vi "ConfigFile_ErrorHandler.vi"(8 "errorArray":errorcluster[](array[cluster]), 9 "foundArray":bool[](array[boolean]), 10 "configItemNameArray":string[](array[string]), 11 "configFilePath (No Path)":path=path "No Path") -> (0 "error out":errorcluster)   [LabVIEW 2024]
doc: "This VI handles errors from reading or writing a configuration file. <B>configFilePath</B> is the path to the configuration file. For the input arrays, all elements must correspond with each other. For example, <B>configItemNameArray[0]</B> is the name of the first configuration item. <B>foundArray[0]</B> is TRUE if the first configuration item was found. <B>errorArray[0]</B> has an error if the read operation for the first configuration item raised an error. <B>error out</B> concatenates all the errors for the configuration arrays into a single error structure."
panel:
  in  "errorCode (9999)":i32=9999
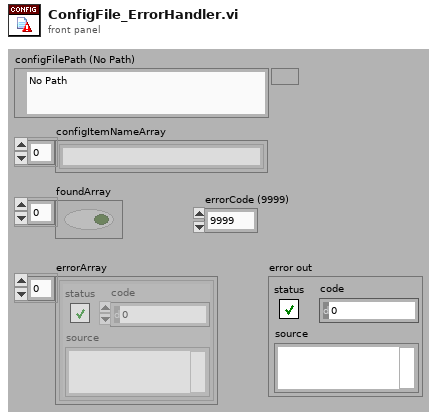
[diagram p1: front panel]
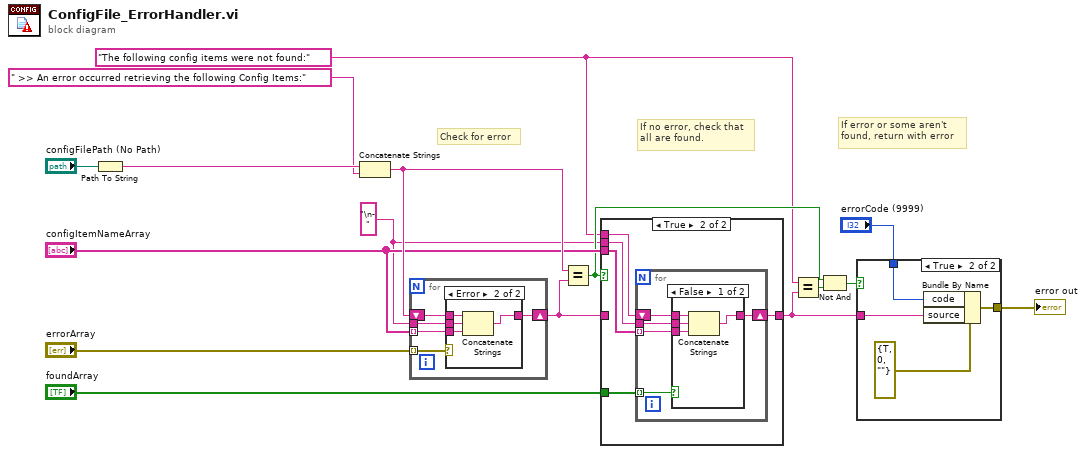
[diagram p0: block diagram]
diagram:
  w6 = "The following config items were not found:"
  w2 = "\n- "
  # "If no error, check that\nall are found."
  # "If error or some aren't\nfound, return with error"
  # "Check for error"
  n1 = Path To String(path="configFilePath (No Path)") -> (string=w15:string)
  n2 = Concatenate Strings(w15, " >> An error occurred retrieving the following Config Items:") -> (w13:string)
  n3 = for {
    tunnel: "errorArray" -> [w21] mode=indexing
    tunnel: "configItemNameArray" -> [w17] mode=indexing
    shift-right: [w20] -> w4
    shift-left: w13 -> [w19]
    tunnel: w2 -> [w18]
    n4 = case shown="Error" w21 {
      tunnel: [w22 w23] -> w20
      tunnel: w19 -> [w22 w26]
      tunnel: w18 -> [_ w25]
      tunnel: w17 -> [_ w24]
      frame No Error {
      }
      frame Error {
        n5 = Concatenate Strings(w26, w25, w24) -> (w23:string)
      }
    }
  }
  n6 = Equal?(x=w13, y=w4) -> (x = y?=w8:bool)
  n7 = case shown="True" w8 {
    tunnel: "foundArray" -> [_ w32]
    tunnel: w4 -> [w27 _]
    tunnel: [w27 w28] -> w5
    tunnel: w6 -> [_ w31]
    tunnel: "configItemNameArray" -> [_ w30]
    tunnel: w2 -> [_ w29]
    frame False {
    }
    frame True {
      n8 = for {
        tunnel: w32 -> [w37] mode=indexing
        tunnel: w30 -> [w33] mode=indexing
        shift-right: [w36] -> w28
        shift-left: w31 -> [w35]
        tunnel: w29 -> [w34]
        n9 = case shown="False" w37 {
          tunnel: [w38 w42] -> w36
          tunnel: w35 -> [w41 w42]
          tunnel: w34 -> [w40 _]
          tunnel: w33 -> [w39 _]
          frame False {
            n10 = Concatenate Strings(w41, w40, w39) -> (w38:string)
          }
          frame True {
          }
        }
      }
    }
  }
  n11 = Equal?(x=w6, y=w5) -> (x = y?=w7:bool)
  n12 = Not And(1:w7, 2:w8) -> (0:w9:bool)
  n13 = case shown="True" w9 {
    tunnel: [_ w46] -> w3
    tunnel: w5 -> [_ w45]
    tunnel: "errorCode (9999)" -> [_ w43]
    frame False {
    }
    frame True {
      n14 = Bundle By Name(cluster=errorcluster {"status"=TRUE, "code"=0, "source"=""} ("error out 2"), "code"=w43, "source"=w45) -> (w46:errorcluster)
    }
  }
  "error out" <- w3
